vi "main.vi"() -> ()   [LabVIEW 2017]
doc: "Demonstrates how to write and receive CAN frames via the Network Interface on the same port. \n\nTo write and receive frames via the Network Interface:\n- select the CAN Network Interface (i.e. CAN0, CAN1, etc.)\n- select the Baud Rate\n- run the VI\n- press the write button to write frames to the can bus\n\nEnable RTR Button to send a Remote Transmission Request or to simply send an empty Frame to request an Answer Frame from a connected device.\n\nEnable Extended Button to write extended Identifier Format. This is done by setting the 30th bit to enable extended format with the driver."
uses:
  <vilib>/nican/nican.llb/CanFrameTimed.ctl
  <vilib>/nican/nican.llb/ncNetAttr.ctl
panel:
  in  "binFile":path=path "C:/Users/twalling/Desktop/hubert-master/hubert-master/examples/02-blinky/Debug/blinky.bin"
  out "msgDataDl":T1[](array[typedef]) {"Data" format="%.0x"; "ArbitrationId" format="%.0x"; "Timestamp" format="%<%I:%M:%S%3u %p\n%m/%d/%Y>T"}
  in  "interface":string(combo)="CAN0" caption="Interface"
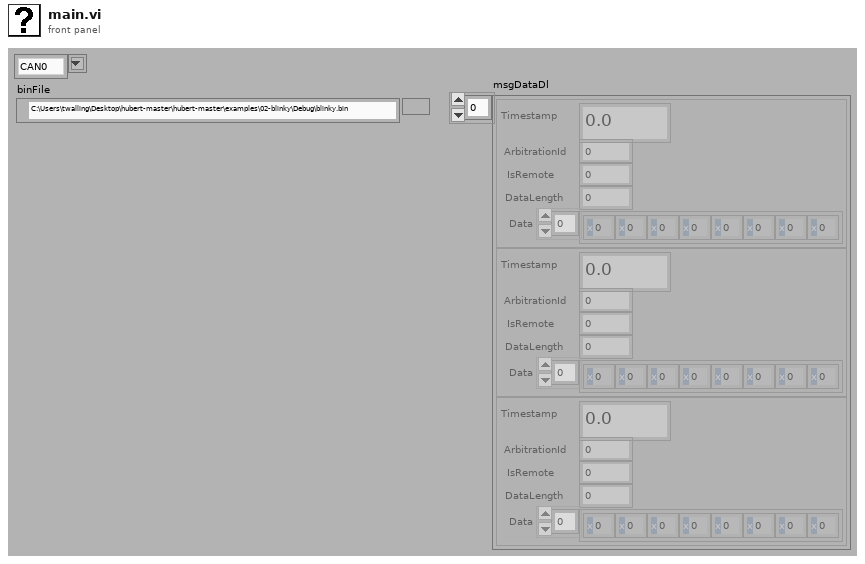
[diagram p1: front panel]
types:
  T1 = typedef "CanFrameTimed.ctl" = cluster{"Timestamp":dbl, "ArbitrationId":u32, "IsRemote":u8, "DataLength":u8, "Data":u8[]}
  T2 = typedef "ncNetAttr.ctl" = cluster{"Start On Open":enum32{"FALSE", "TRUE"}, "Baud Rate":u32, "Read Queue Length":u32, "Write Queue Length":u32, "Standard Comparator":u32, "Standard Mask":u32, "Extended Comparator":u32, "Extended Mask":u32}
  T3 = typedef "xobjhandle.ctl" = u32
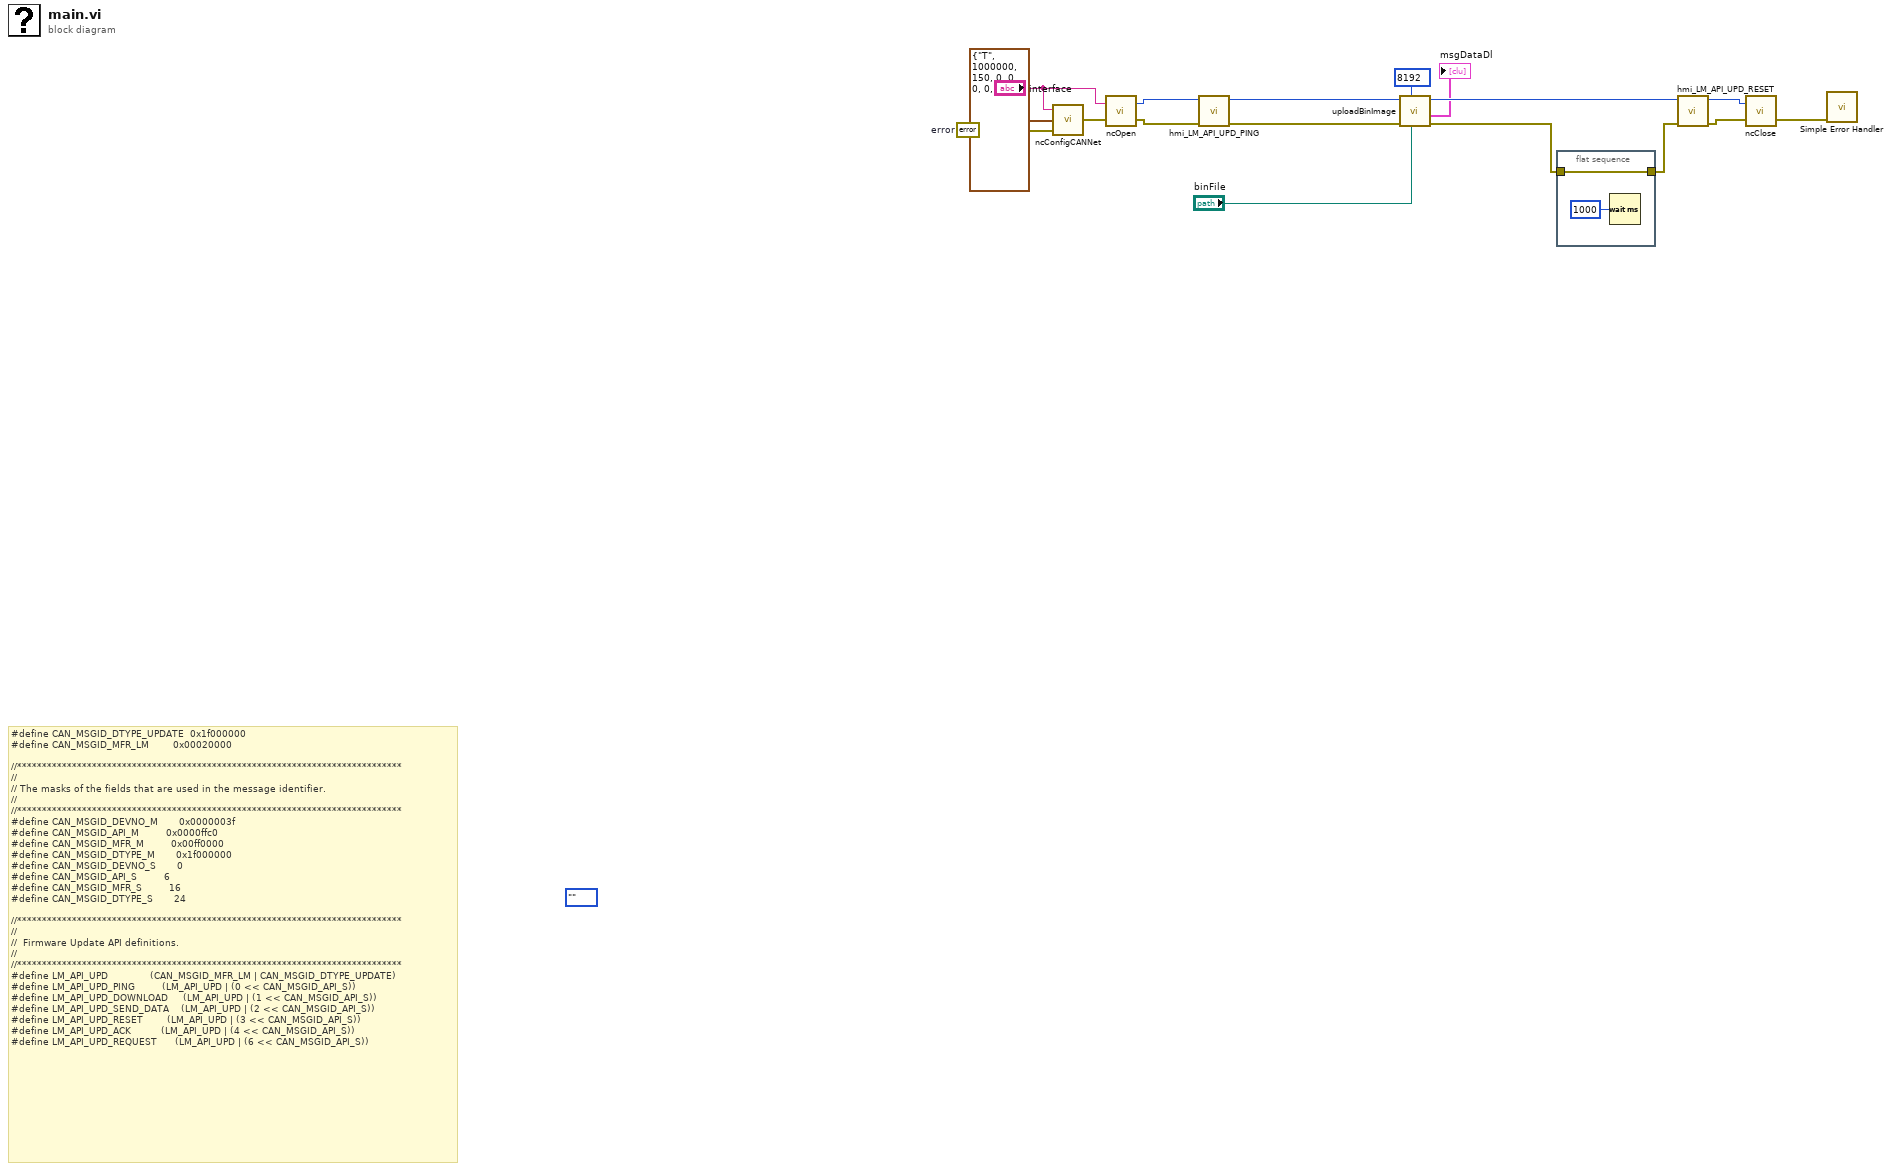
[diagram p0: block diagram]
diagram:
  (unwired) enum32{""}.""
  w15 = errorcluster {"status"=FALSE, "code"=0, "source"=""}  # error
  # "#define CAN_MSGID_DTYPE_UPDATE  0x1f000000\n#define CAN_MSGID_MFR_LM        0x00020000\n\n//*****************************************************************************\n//\n// The masks of the fields that are used in the message identifier.\n//\n//*****************************************************************************\n#define CAN_MSGID_DEVNO_M       0x0000003f\n#define CAN_MSGID_API_M         0x0000ffc0\n#define CAN_MSGID_MFR_M         0x00ff0000\n#define CAN_MSGID_DTYPE_M       0x1f000000\n#define CAN_MSGID_DEVNO_S       0\n#define CAN_MSGID_API_S         6\n#define CAN_MSGID_MFR_S         16\n#define CAN_MSGID_DTYPE_S       24\n\n//*****************************************************************************\n//\n//  Firmware Update API definitions.\n//\n//*****************************************************************************\n#define LM_API_UPD              (CAN_MSGID_MFR_LM | CAN_MSGID_DTYPE_UPDATE)\n#define LM_API_UPD_PING         (LM_API_UPD | (0 << CAN_MSGID_API_S))\n#define LM_API_UPD_DOWNLOAD     (LM_API_UPD | (1 << CAN_MSGID_API_S))\n#define LM_API_UPD_SEND_DATA    (LM_API_UPD | (2 << CAN_MSGID_API_S))\n#define LM_API_UPD_RESET        (LM_API_UPD | (3 << CAN_MSGID_API_S))\n#define LM_API_UPD_ACK          (LM_API_UPD | (4 << CAN_MSGID_API_S))\n#define LM_API_UPD_REQUEST      (LM_API_UPD | (6 << CAN_MSGID_API_S))"
  n1 = call <vilib>:"ncConfigCANNet.vi"("Error in"=w15, "CAN Network Interface Config"=T2 {"Start On Open"=enum."TRUE", "Baud Rate"=1000000, "Read Queue Length"=150, "Write Queue Length"=0, "Standard Comparator"=0, "Standard Mask"=0, "Extended Comparator"=0, "Extended Mask"=0}, "ObjName"="interface") -> ("Error out"=w16:errorcluster)  [unwired: 2 in]
  n2 = call <vilib>:"ncOpen.vi"("Error in"=w16, "ObjName"="interface") -> ("Error out"=w11:errorcluster, "ObjHandle out"=w12:T3)
  n3 = call "hmi_LM_API_UPD_PING.vi"("Error in"=w11, "canSession"=w12) -> ("Error out"=w6:errorcluster, "canSession"=w7:T3)  [unwired: 7 in, 1 out]
  n4 = call "uploadBinImage.vi"("binFile"="binFile", "dloadAddr"=u32 8192 ("dloadSize"), "Error in"=w6, "canSession"=w7) -> ("Error out"=w5:errorcluster, "msgData"=→"msgDataDl":T1[], "canSession"=w4:T3)  [unwired: 5 in]
  n5 = flat-sequence {
    tunnel: w5 -> [w19]
    tunnel: [w19] -> w8
    frame #0 {
      n6 = Wait (ms)(milliseconds to wait=u32 1000) -> ()  [unwired: 1 out]
    }
  }
  n7 = call "hmi_LM_API_UPD_RESET.vi"("Error in"=w8, "canSession"=w4) -> ("Error out"=w10:errorcluster, "canSession"=w9:T3)  [unwired: 8 in]
  n8 = call <vilib>:"ncClose.vi"("Error in"=w10, "ObjHandle in"=w9) -> ("Error out"=w13:errorcluster)  [unwired: 1 in]
  n9 = call <vilib>:"Simple Error Handler.vi"("error in (no error)"=w13) -> ()  [unwired: 4 in, 5 out]
